vi "Label Targets3.vi"(8 "Score Threshold":dbl=75.0, 9 "Annotate":bool=TRUE, 10 "Targets":T2(array[cluster]), 11 "Image in":T1) -> (3 "Image out":T1)   [LabVIEW 2025]
doc: "Draw text scores near or on the particle. Scores above the limit are green and underlined."
uses:
  <vilib>/vision/Image Controls.llb/IMAQ Image.ctl
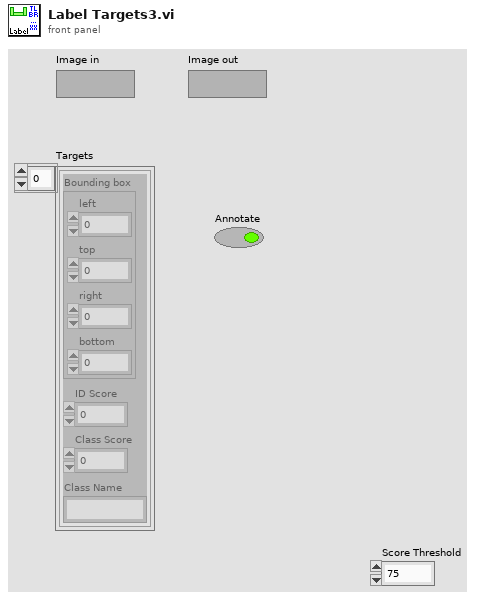
[diagram p1: front panel]
types:
  T1 = typedef "IMAQ Image.ctl" = refnum<image>
  T2 = cluster{"Bounding box":cluster{"left":dbl, "top":dbl, "right":dbl, "bottom":dbl}, "ID Score":dbl, "Class Score":dbl, "Class Name":string}[]
  T3 = cluster{"Desired Font (Application)":enum16{"User-specified Font", "Application Font", "System Font", "Dialog Font"}, "[User-specified Font]":cluster{"Font Name":string, "Size":i16, "Strikeout?":bool, "Italic?":bool, "Underline?":bool, "Outline?":bool, "Shadow?":bool, "Bold?":bool, "Rotation Angle":dbl}, "Horizontal Alignment":i16, "Vertical Alignment":i16}
  T4 = cluster{"left":dbl, "top":dbl, "right":dbl, "bottom":dbl}
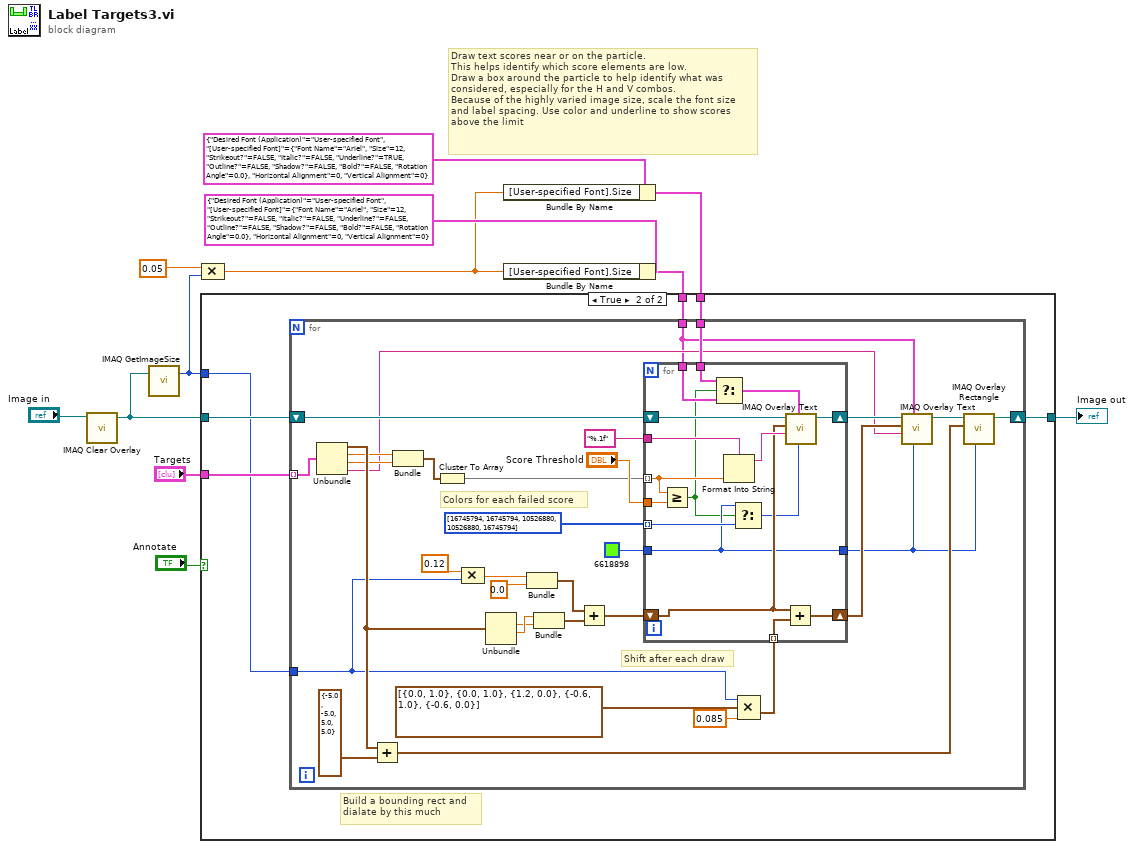
[diagram p0: block diagram]
diagram:
  # "Draw text scores near or on the particle.\nThis helps identify which score elements are low.\nDraw a box around the particle to help identify what was\nconsidered, especially for the H and V combos.\nBecause of the highly varied image size, scale the font size\nand label spacing. Use color and underline to show scores\nabove the limit"
  n1 = call "IMAQ Clear Overlay"("Image"="Image in") -> ("Image Out"=w4:T1)  [unwired: 2 in, 8 out]
  n2 = call "IMAQ GetImageSize"("Image"=w4) -> ("Y Resolution"=w3:i32)  [unwired: 3 in, 2 out]
  n3 = Compound Arithmetic op=MULTIPLY(0.05, w3) -> (w2:dbl)
  n4 = Bundle By Name(cluster=T3 {"Desired Font (Application)"=enum."User-specified Font", "[User-specified Font]"={"Font Name"="Ariel", "Size"=12, "Strikeout?"=FALSE, "Italic?"=FALSE, "Underline?"=TRUE, "Outline?"=FALSE, "Shadow?"=FALSE, "Bold?"=FALSE, "Rotation Angle"=0.0}, "Horizontal Alignment"=0, "Vertical Alignment"=0} ("Font, Size & Style"), "[User-specified Font].Size"=w2) -> (w5:T3)
  n5 = Bundle By Name(cluster=T3 {"Desired Font (Application)"=enum."User-specified Font", "[User-specified Font]"={"Font Name"="Ariel", "Size"=12, "Strikeout?"=FALSE, "Italic?"=FALSE, "Underline?"=FALSE, "Outline?"=FALSE, "Shadow?"=FALSE, "Bold?"=FALSE, "Rotation Angle"=0.0}, "Horizontal Alignment"=0, "Vertical Alignment"=0} ("Font, Size & Style"), "[User-specified Font].Size"=w2) -> (w6:T3)
  n6 = case shown="True" "Annotate" {
    tunnel: [w13 w19] -> w12
    tunnel: "Targets" -> [_ w18]
    tunnel: w4 -> [w13 w17]
    tunnel: w5 -> [_ w16]
    tunnel: w6 -> [_ w15]
    tunnel: w3 -> [_ w14]
    frame False {
    }
    frame True {
      # "Build a bounding rect and\ndialate by this much"
      n7 = for {
        tunnel: w18 -> [w47] mode=indexing
        shift-right: [w48] -> w19
        shift-left: w17 -> [w52]
        tunnel: w14 -> [w27]
        tunnel: w16 -> [w31]
        tunnel: w15 -> [w21]
        # "Colors for each failed score"
        # "Shift after each draw"
        n8 = Unbundle(w47) -> ("Bounding box"=w41:T4, "ID Score"=w39:dbl, "Class Score"=w38:dbl, "Class Name"=w22:string)
        n9 = Add(x=w41, y=cluster{dbl, dbl, dbl, dbl} {-5.0, -5.0, 5.0, 5.0} ("output cluster")) -> (x+y=w43:cluster{dbl, dbl, dbl, dbl})
        n10 = Bundle("ID Score"=w39, "Class Score"=w38) -> (w49:cluster{"ID Score":dbl, "Class Score":dbl})  [unwired: 1 in]
        n11 = Cluster To Array(cluster=w49) -> (array=w40:dbl[])
        n12 = Compound Arithmetic op=MULTIPLY(0.12, w27) -> (w28:dbl)
        n13 = Unbundle(w41) -> ("top"=w45:dbl, "right"=w46:dbl)  [unwired: 2 out]
        n14 = Bundle(w28, 0.0) -> (w30:cluster{dbl, dbl})  [unwired: 1 in]
        n15 = Bundle("right"=w46, "top"=w45) -> (w44:cluster{"right":dbl, "top":dbl})  [unwired: 1 in]
        n16 = Add(x=w30, y=w44) -> (x+y=w51:cluster{dbl, dbl})
        n17 = Compound Arithmetic op=MULTIPLY(w27, cluster{dbl, dbl}[] [{0.0, 1.0}, {0.0, 1.0}, {1.2, 0.0}, {-0.6, 1.0}, {-0.6, 0.0}], 0.085) -> (w35:cluster{dbl, dbl}[])
        n18 = for {
          tunnel: w40 -> [w62] mode=indexing
          shift-right: [w65] -> w23
          shift-left: w51 -> [w64]
          shift-right: [w66] -> w25
          shift-left: w52 -> [w67]
          tunnel: u32[] [16745794, 16745794, 10526880, 10526880, 16745794] -> [w63] mode=indexing
          tunnel: "Score Threshold" -> [w61]
          tunnel: w35 -> [w59] mode=indexing
          tunnel: "%.1f" ("format string") -> [w58]
          tunnel: u32 6618898 ("Color") -> [w57]
          tunnel: [w57] -> w20
          tunnel: w31 -> [w56]
          tunnel: w21 -> [w55]
          n19 = Greater Or Equal?(x=w62, y=w61) -> (x >= y?=w54:bool)
          n20 = Select(t=w56, s=w54, f=w55) -> (s? t:f=w53:T3)
          n21 = Format Into String(format string=w58, w62) -> (resulting string=w68:string)  [unwired: 2 in, 1 out]
          n22 = Select(t=w57, s=w54, f=w63) -> (s? t:f=w60:u32)
          n23 = Add(x=w59, y=w64) -> (x+y=w65:cluster{dbl, dbl})
          n24 = call "IMAQ Overlay Text"("Text Color (black)"=w60, "Font, Size & Style"=w53, "String"=w68, "Origin"=w64, "Image"=w67) -> ("Image Out"=w66:T1)  [unwired: 5 in, 1 out]
        }
        n25 = call "IMAQ Overlay Text"("Text Color (black)"=w20, "Font, Size & Style"=w21, "String"=w22, "Origin"=w23, "Image"=w25) -> ("Image Out"=w24:T1)  [unwired: 5 in, 1 out]
        n26 = call "IMAQ Overlay Rectangle"("Color"=w20, "Rectangle"=w43, "Image"=w24) -> ("Image Out"=w48:T1)  [unwired: 7 in, 1 out]
      }
    }
  }
  "Image out" <- w12
